vi "LRem.vi"(0 "reference in":refnum<class "Redis.lvclass">, 1 "Key":string, 7 "Count":i32, 9 "Element":string, 11 "Error In":errorcluster) -> (4 "reference out":refnum<class "Redis.lvclass">, 8 "Return":i64, 15 "Error Out":errorcluster)   [LabVIEW 2020, in "Redis.lvclass"]
doc: "<b>LREM</b>\n\nRemoves the first count occurrences of elements equal to element from the list stored at key. The count argument influences the operation in the following ways:\n\ncount > 0: Remove elements equal to element moving from head to tail.\ncount < 0: Remove elements equal to element moving from tail to head.\ncount = 0: Remove all elements equal to element.\nFor example, LREM list -2 \"hello\" will remove the last two occurrences of \"hello\" in the list stored at list.\n\nNote that non-existing keys are treated like empty lists, so when key does not exist, the command will always return 0."
uses:
  Redis.lvclass
  Redis.lvclass/Redis.ctl
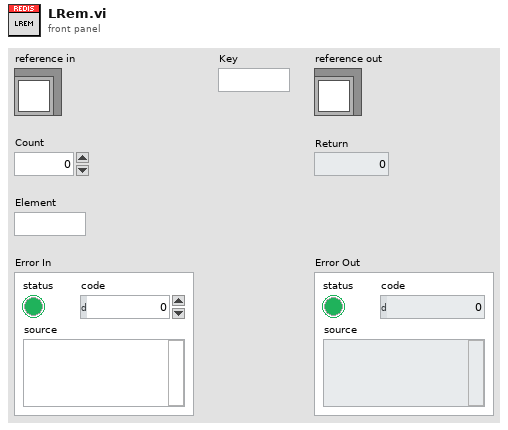
[diagram p1: front panel]
types:
  T1 = typedef "Redis.lvclass/RedisDataType.ctl" = cluster{"Reply Type":T2, "Integer":i64, "String":string, "Multibulk":variant[], "StringData":string[]}
  T2 = typedef "Redis.lvclass/ReplyDataTypeEnum.ctl" = enum16{"None", "Error", "Status", "Nil", "Integer", "String", "Multibulk"}
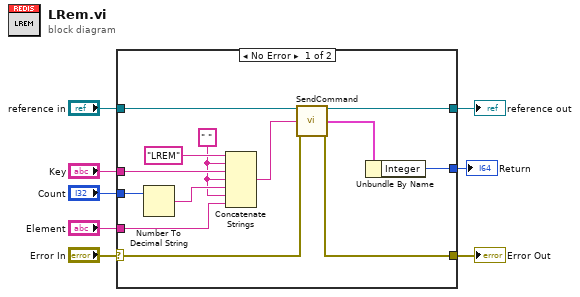
[diagram p0: block diagram]
diagram:
  n1 = case shown="No Error" "Error In" {
    selector: "Error In" -> [w19 w23]
    tunnel: [w18 w23] -> w7
    tunnel: [w21 w22] -> w5
    tunnel: "reference in" -> [w20 w22]
    tunnel: "Key" -> [w16 _]
    tunnel: "Count" -> [w14 _]
    tunnel: [w11 _] -> w1
    tunnel: "Element" -> [w9 _]
    frame No Error {
      w10 = " "
      n2 = Number To Decimal String(number=w14) -> (decimal integer string=w13:string)  [unwired: 1 in]
      n3 = Concatenate Strings("LREM", w10, w16, w10, w13, w10, w9) -> (w15:string)
      n4 = call "SendCommand.vi"("reference in"=w20, "Command"=w15, "Error In"=w19) -> ("reference out"=w21:refnum<class "Redis.lvclass">, "Data"=w12:T1, "Error Out"=w18:errorcluster)  [unwired: 10 in]
      n5 = Unbundle By Name(w12) -> ("Integer"=w11:i64)
    }
    frame Error {
    }
  }
  "Error Out" <- w7
  "reference out" <- w5
  "Return" <- w1
